vi "Filter and Log Error.vi"(8 "error In":errorcluster) -> ()   [LabVIEW 2021, in "CIFPluginManager.lvclass"]
uses:
  CIFPluginManager.lvclass
  CIFPluginManager.lvclass/CIFPluginManager.ctl
  CIFUtilities/CIFLogs/CIFLogs.lvlib
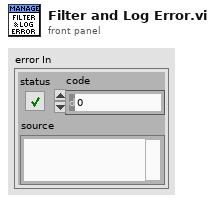
[diagram p1: front panel]
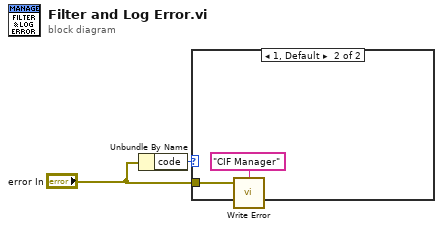
[diagram p0: block diagram]
diagram:
  n1 = Unbundle By Name("error In") -> ("code"=w2:i32)
  n2 = case shown="1, Default" w2 {
    tunnel: "error In" -> [_ w4]
    frame -1001, -2, 0 {
      # "-1001 is cancelled by client.  Not an error.\n-2 (Invalid Argument) can be caused by race condition on client timeout."
    }
    frame 1, Default {
      n3 = call "Write Error.vi"("error in (no error)"=w4, "Plugin Name"="CIF Manager") -> ()  [unwired: 2 in, 1 out]
    }
  }
